vi "Save_Picture_Parameter_FGV.vi"(8 "error in":errorcluster, 10 "FGV_Control":enum16{"Set", "Get"}(ring), 11 "Picture_Parameter_In":T2) -> (0 "error out":errorcluster, 3 "Picture_Parameter_Out":T1)   [LabVIEW 2011]
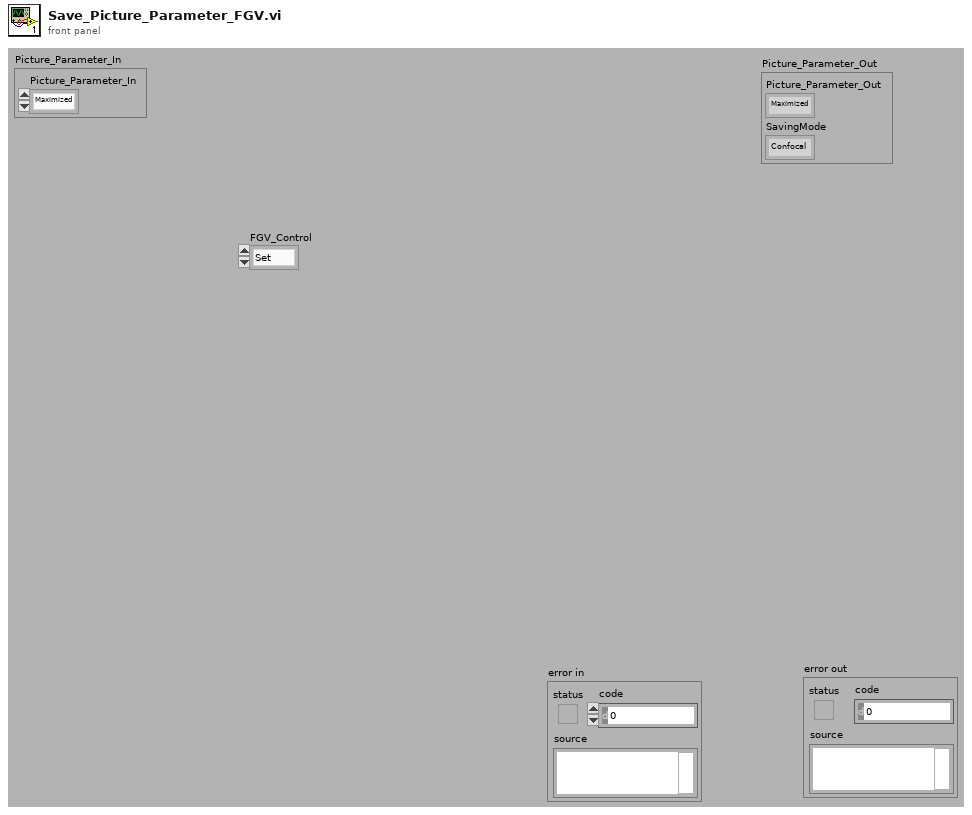
[diagram p1: front panel]
types:
  T1 = cluster{"Picture_Parameter_Out":enum16{"Maximized", "Averaged", "Normalized"}, "SavingMode":enum32{"Confocal", "HighRes", "Video", "Picture", "IntensityTrace", "Test"}}
  T2 = cluster{"Picture_Parameter_In":enum16{"Maximized", "Averaged", "Normalized"}}
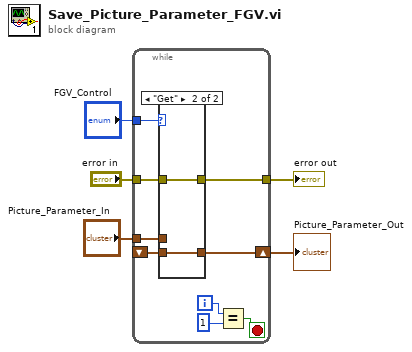
[diagram p0: block diagram]
diagram:
  n1 = while {
    tunnel: "Picture_Parameter_In" -> [w14]
    shift-right: [w13] -> w1
    shift-left: _ -> [w12]
    tunnel: "error in" -> [w8]
    tunnel: [w7] -> w4
    tunnel: "FGV_Control" -> [w6]
    i -> [w9]
    stop <- w10 stop-if-true
    n2 = case shown="\"Get\"" w6 {
      tunnel: w14 -> [w16 _]
      tunnel: [w16 w18] -> w13
      tunnel: w12 -> [_ w18]
      tunnel: w8 -> [w15 w17]
      tunnel: [w15 w17] -> w7
      frame "Set", Default {
      }
      frame "Get" {
      }
    }
    n3 = Equal?(x=w9, y=1) -> (x = y?=w10:bool)
  }
  "error out" <- w4
  "Picture_Parameter_Out" <- w1
